vi "Item_OnPopupMenu.vi"(11 "Object":T1) -> ()   [LabVIEW 2020, in "Message Rescripter.lvlib"]
uses:
  Message Rescripter.lvlib
  <resource>/Framework/Providers/API/mxLvMenuItem.ctl
  Support/Localized Strings.vi
  MessageMakerProvider/AFPP Shared/Validation Mode.ctl
  MessageMakerProvider/AFPP Shared/AFPP Shared.lvlib
  <resource>/Framework/Providers/API/ItemRef.ctl
panel:
  out "error out":errorcluster
  in  "error in":errorcluster
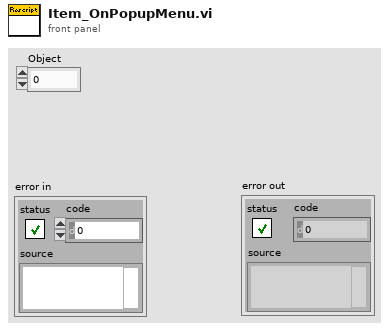
[diagram p1: front panel]
types:
  T1 = typedef "ItemRef.ctl" = u64
  T2 = typedef "AFPP Shared.lvlib/Validation Mode.ctl" = enum16{"An Actor Library", "A Target Tag"}
  T3 = typedef "mxLvMenuItem.ctl" = cluster{"Menu Name":string, "Description":string, "Icon File Name":path, "Menu Tag":string, "Enabled":bool, "Checked":bool, "Separator":bool, "Batchable":bool, "Weight":i32, "Batch Mode (Ignored if Not Batchable)":enum32{"Show If All Items Support Command", "Show If Any Items Support Command"}, "Menu Location":enum32{"<None>", "Project", "Project / Build Specifications", "Tools", "Tools / Source Control", "Tools / Real-Time Module", "Help"}, "Exclude From Getting Started Window Menu":bool}
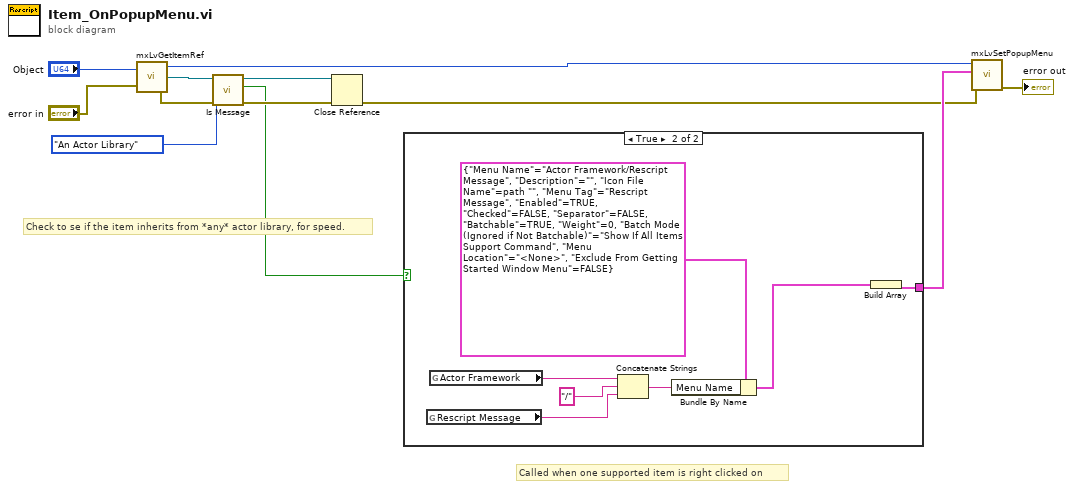
[diagram p0: block diagram]
diagram:
  # "Check to se if the item inherits from *any* actor library, for speed."
  # "Called when one supported item is right clicked on"
  n1 = call <resource>:"mxLvGetItemRef.vi"("Item"="Object", "error in"="error in") -> ("Item"=w11:T1, "Item Refnum"=w8:refnum<vi>, "error out"=w4:errorcluster)
  n2 = call "Is Message.vi"("error in (no error)"=w4, "Validation"=Validation_Mode."An Actor Library", "ProjectItem in"=w8) -> ("error out"=w5:errorcluster, "Is Message"=w3:bool, "ProjectItem out"=w6:refnum<vi>)  [unwired: 6 in]
  n3 = Close Reference(reference=w6, error in (no error)=w5) -> (error out=w2:errorcluster)
  n4 = case shown="True" w3 {
    tunnel: [_ w17] -> w10
    frame False {
    }
    frame True {
      n5 = global read "Localized Strings.vi" "Rescript Message"() -> (w13:string)
      n6 = global read "Localized Strings.vi" "Actor Framework"() -> (w14:string)
      n7 = Concatenate Strings(w14, "/", w13) -> (w16:string)
      n8 = Bundle By Name(cluster=T3 {"Menu Name"="Actor Framework/Rescript Message", "Description"="", "Icon File Name"=path "", "Menu Tag"="Rescript Message", "Enabled"=TRUE, "Checked"=FALSE, "Separator"=FALSE, "Batchable"=TRUE, "Weight"=0, "Batch Mode (Ignored if Not Batchable)"=enum."Show If All Items Support Command", "Menu Location"=enum."<None>", "Exclude From Getting Started Window Menu"=FALSE} ("Menu Item"), "Menu Name"=w16) -> (w18:T3)
      n9 = Build Array(w18) -> (w17:T3[])
    }
  }
  n10 = call <resource>:"mxLvSetPopupMenu.vi"("error in"=w2, "Popup Menu Items"=w10, "Item"=w11) -> ("error out"=→"error out":errorcluster)  [unwired: 7 in, 1 out]
